vi "Shutdown.vi"(8 "error in":errorcluster, 11 "objects in":T1) -> (0 "error out":errorcluster, 3 "objects out":T1)   [LabVIEW 2011]
uses:
  Controls/Class Objects.ctl
  Modules/File/Configuration/Configuration.lvclass
  Modules/Hardware/Power Supply/Power Supply.lvclass
  Modules/Hardware/Mass Flow Controller/Mass Flow Controller.lvclass
  Modules/File/TDMS/TDMS.lvclass
  Controls/Class Labels.ctl
  Controls/User Interface Action.ctl
  Modules/Menu/Menu Action.ctl
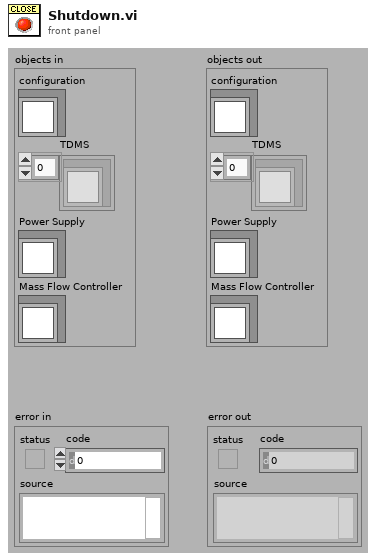
[diagram p1: front panel]
types:
  T1 = typedef "Class Objects.ctl" = cluster{"configuration":refnum<class "Configuration.lvclass">, "TDMS":refnum<class "TDMS.lvclass">[], "Power Supply":refnum<class "Power Supply.lvclass">, "Mass Flow Controller":refnum<class "Mass Flow Controller.lvclass">}
  T2 = typedef "Class Labels.ctl" = enum16{"Configuration", "TDMS", "PID", "Power Supply", "Vapour Generator", "MFC", "NMR", "Valve Controller", "Multimeter"}
  T3 = typedef "User Interface Action.ctl" = enum16{"Initialize", "Visibility Front Panel Controls", "Stop"}
  T4 = typedef "Menu Action.ctl" = enum16{"Initialize", "Insert Item", "Remove Item", "Set Checked Item", "Get Checked Item", "Get Item Index", "Item Present?", "Stop"}
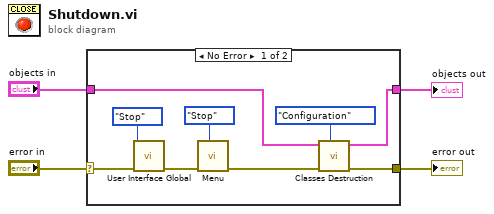
[diagram p0: block diagram]
diagram:
  n1 = case shown="No Error" "error in" {
    selector: "error in" -> [w12 w15]
    tunnel: [w7 w15] -> w3
    tunnel: "objects in" -> [w6 w14]
    tunnel: [w5 w14] -> w1
    frame No Error {
      n2 = call "User Interface Global.vi"("error in"=w12, "action"=User_Interface_Action."Stop") -> ("error out"=w11:errorcluster)  [unwired: 9 in]
      n3 = call "Menu.vi"("action"=Menu_Action."Stop" ("Menu"), "error in"=w11) -> ("error out"=w8:errorcluster)  [unwired: 6 in, 3 out]
      n4 = call "Classes Destruction.vi"("class labels"=Class_Labels."Configuration", "error in"=w8, "classes in"=w6) -> ("error out"=w7:errorcluster, "classes out"=w5:T1)  [unwired: 7 in]
    }
    frame Error {
    }
  }
  "error out" <- w3
  "objects out" <- w1
